vi "Async 985x Incoming Engine.vi"() -> ()   [LabVIEW 2020, in "985x Support Addon Engine.lvlib"]
uses:
  985x Support Addon Engine.lvlib
  <vilib>/NI/NIVS Inline Async API/_VS Inline Async API/Process/Process.lvclass
  Addon/Addon Engine/Types/RT Async Engine Settings.ctl
  Addon/Addon Shared/Types/XNET Settings.ctl
  Frame-Protection-Support/Source/Engine/Types/RT Frame Settings.ctl
  Frame-Protection-Support/Source/Shared/Types/Exported Frame Type.ctl
  Frame-Protection-Support/Source/Engine/Types/RT Protection Configuration.ctl
  Frame-Protection-Support/Source/Shared/Types/Protection Type.ctl
  Frame-Protection-Support/Source/Shared/Types/XNET Signal Configuration.ctl
  Frame-Protection-Support/Source/Shared/Types/Exported Counter Settings.ctl
  Frame-Protection-Support/Source/Shared/Types/Exported Event Trigger Type.ctl
  Frame-Protection-Support/Source/Engine/Types/RT Frame Incoming Values.ctl
  Types/985x Settings.ctl
  Types/FPGA Refnum.ctl
  <vilib>/NI/NIVS Inline Async API/_VS Inline Async API/Process/Process.lvclass/Process.ctl
  <vilib>/NI/NIVS Inline Async API/_VS Inline Async API/Error Handling Process/SubVIs/Error.ConvertArray.vi
  <vilib>/rvi/interface/common/niFpgaWaitOnOcc.vi
  <vilib>/Utility/error.llb/Error Cluster From Error Code.vi
  <vilib>/rvi/errors/niLvFpgaAdjustHostInterfaceError.vi
  985x Properties.vi
  <vilib>/rvi/interface/nirviMethod/nirviMethod.xnode
  <vilib>/rvi/errors/niLvFpgaMergeErrorWithErrorCode.vi
  <vilib>/FPGAPlugInAG/Dynamic/niLvFpga_AcknowledgeIrq_Dynamic.vi
  <vilib>/FPGAPlugInAG/Dynamic/niLvFpga_ReadFifo_Dynamic.vi
  Frame-Protection-Support/Source/Engine/Protection and Counter Support Engine.lvlib
  Frame-Protection-Support/Source/Shared/Protection and Counter Support Shared.lvlib
  Addon/Addon Shared/Protection and Counter Addon Shared.lvlib
  Addon/Addon Engine/Protection and Counter Addon Engine.lvlib
  <vilib>/FPGAPlugInAG/Dynamic/niLvFpga_ConfigureFifo_Dynamic.vi
  <vilib>/FPGAPlugInAG/Dynamic/niLvFpga_StartFifo_Dynamic.vi
panel:
  in  "Parameters":variant
  in  "Process":refnum<class "Process.lvclass">
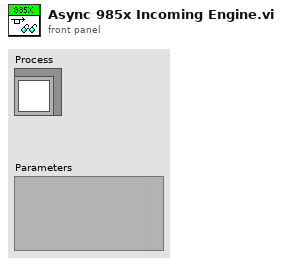
[diagram p1: front panel]
types:
  T1 = enum16{"open", "replace", "create", "open or create", "replace or create", "replace or create with confirmation"}
  T2 = typedef "Protection and Counter Addon Engine.lvlib/RT Async Engine Settings.ctl" = cluster{"Name":string, "Priority":i32, "XNET Settings":T3, "FPGA Session":u32, "Outgoing CAN Session":refnum<k21>, "Outgoing Frame Count":i32, "Outgoing Frames":T4[], "Incoming CAN Session":refnum<k21>, "Incoming Frame Count":i32, "Incoming Frames":T4[], "Incoming Values":T11, "985x Settings":T12}
  T3 = typedef "Protection and Counter Addon Shared.lvlib/XNET Settings.ctl" = cluster{"Database":refnum<k21>, "Cluster":refnum<k21>, "Port":string, "Baud rate [Bd]":u64, "Termination":u32, "CAN I/O Mode":u32, "FD Baud rate [Bd]":u64, "Priority":i32, "Use Legacy":bool, "FD ISO Mode":u32}
  T4 = typedef "Protection and Counter Support Engine.lvlib/RT Frame Settings.ctl" = cluster{"Type":T5, "Frame ID":u32, "Payload Length":u32, "VS Offset":i32, "VS Length":i32, "Frame Conversion":refnum<k21>, "Frame.Data":dbl[], "Generation Period":u32, "Time Since Last Generation":u32, "Generation Iterations":u32, "Generation Counter":u32, "Has Protection?":bool, "Protection Configurations":T6[], "Has Counter?":bool, "Counter Configurations":T9[], "Has Disable?":bool, "Disable VS Index":i32, "Transmit Trigger":T10, "Trigger VS Index":i32}
  T5 = typedef "Protection and Counter Support Shared.lvlib/Exported Frame Type.ctl" = enum16{"Periodic", "Event", "Periodic/Event"}
  T6 = typedef "Protection and Counter Support Engine.lvlib/RT Protection Configuration.ctl" = cluster{"Protection Frame Index":i32, "Protection Type":T7, "Data Indeces":i32[], "Data Array":dbl[], "Check Sum Conversion":refnum<k21>, "CRC Channels":T8[], "Protection VS Index":i32, "Counter Data Index":i32, "Override Index":i32, "Override Value Index":i32}
  T7 = typedef "Protection and Counter Support Shared.lvlib/Protection Type.ctl" = enum16{"Arb ID + Bytes Checksum with Inversion", "Arb ID + Bytes CRC with Inversion", "Reversed Raw Signal Checksum with Inversion", "Concatenated Two's Compliment"}
  T8 = typedef "Protection and Counter Support Shared.lvlib/XNET Signal Configuration.ctl" = cluster{"Start Bit":i32, "Name":string, "Number of bits":i32, "Scale":dbl, "Offset":dbl, "Data Type":u32, "Counter":bool}
  T9 = typedef "Protection and Counter Support Shared.lvlib/Exported Counter Settings.ctl" = cluster{"Frame Index":i32, "Max Count":dbl, "VS Index":i32, "Bit Length":i64, "Override Index":i32, "Override Value Index":i32}
  T10 = typedef "Protection and Counter Support Shared.lvlib/Exported Event Trigger Type.ctl" = enum16{"Channel value change", "Trigger channel (not zero)", "Channel value change or trigger channel (not zero)", "Trigger channel (any value change)", "Channel value change or trigger channel (any value change)"}
  T11 = typedef "Protection and Counter Support Engine.lvlib/RT Frame Incoming Values.ctl" = cluster{"Signal Values":dbl[], "Signal Invalid Values":dbl[], "ProtCtr Sig Values":dbl[], "Timestamps":timestamp[], "Time Differences":dbl[], "IDs":u32[]}
  T12 = typedef "985x Support Addon Engine.lvlib/985x Settings.ctl" = cluster{"Enable":bool, "FPGA Refnum":T13, "Channel Number":u32, "Rx FIFO":refnum<k33>}
  T13 = typedef "985x Support Addon Engine.lvlib/FPGA Refnum.ctl" = refnum<k20>
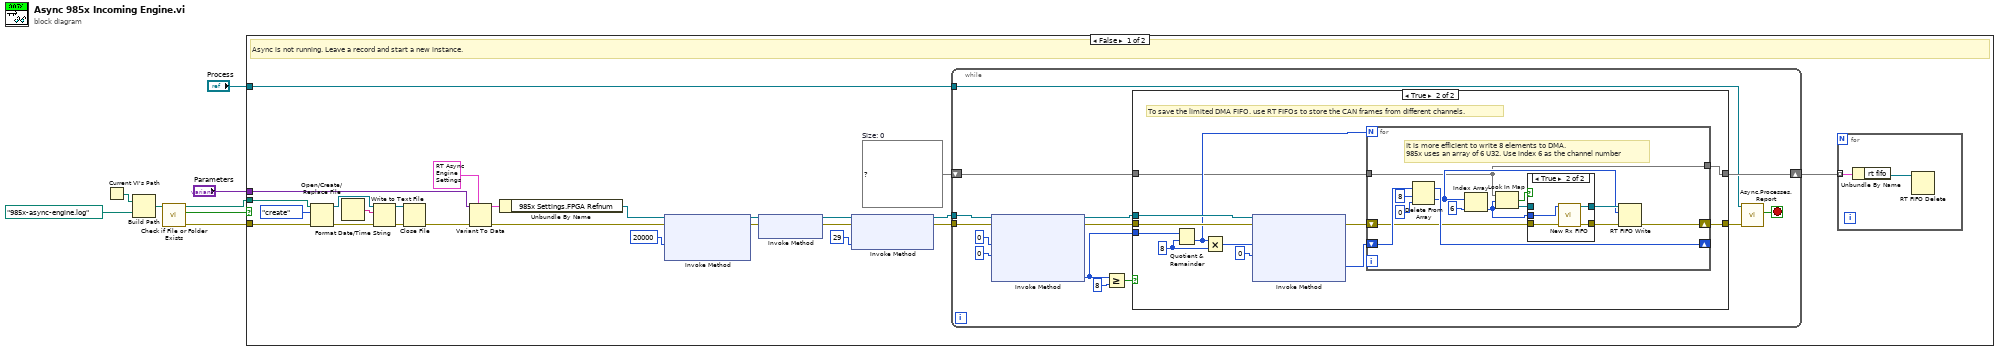
[diagram p0: block diagram]
diagram:
  n1 = Current VI's Path() -> (path=w7:path)
  n2 = Build Path(base path=w7, name or relative path=path "985x-async-engine.log") -> (appended path=w5:path)
  n3 = call <vilib>:"Check if File or Folder Exists.vi"("path"=w5) -> ("error out"=w3:errorcluster, "file or folder exists?"=w2:bool, "dup path"=w4:path)  [unwired: 8 in]
  n4 = case shown="False" w2 {
    tunnel: "Parameters" -> [w23 _]
    tunnel: w4 -> [w14 _]
    tunnel: w3 -> [w13 _]
    tunnel: "Process" -> [w10 _]
    frame False {
      w25 = map{u32, refnum<k33>} {}  # Size: 0
      # "Async is not running. Leave a record and start a new instance."
      n5 = Open/Create/Replace File(file path (use dialog)=w14, error in=w13, operation (0:open)=T1."create") -> (refnum out=w19:refnum<file>, error out=w18:errorcluster)  [unwired: 3 in, 1 out]
      n6 = Format Date/Time String() -> (date/time string=w15:string)  [unwired: 3 in]
      n7 = Write to Text File(file (use dialog)=w19, text=w15, error in=w18) -> (refnum out=w17:refnum<file>, error out=w16:errorcluster)  [unwired: 1 in, 1 out]
      n8 = Close File(refnum=w17, error in=w16) -> (error out=w11:errorcluster)  [unwired: 1 out]
      n9 = Variant To Data(error in=w11, type=T2 {"Name"="", "Priority"=100, "XNET Settings"={"Database"="", "Cluster"="", "Port"="", "Baud rate [Bd]"=0, "Termination"=0, "CAN I/O Mode"=0, "FD Baud rate [Bd]"=500000, "Priority"=100, "Use Legacy"=FALSE, "FD ISO Mode"=0}, "FPGA Session"=0, "Outgoing CAN Session"="", "Outgoing Frame Count"=0, "Outgoing Frames"=[], "Incoming CAN Session"="", "Incoming Frame Count"=0, "Incoming Frames"=[], "Incoming Values"={"Signal Values"=[], "Signal Invalid Values"=[], "ProtCtr Sig Values"=[], "Timestamps"=[], "Time Differences"=[], "IDs"=[]}, "985x Settings"={"Enable"=FALSE, "FPGA Refnum"=refnum, "Channel Number"=0, "Rx FIFO"=refnum}} ("RT Configuration"), Variant=w23) -> (data=w21:T2, error out=w22:errorcluster)
      n10 = Unbundle By Name(w21) -> ("985x Settings.FPGA Refnum"=w20:T13)
      n11 = xnode "Invoke Method"("FPGA VI Reference In"=w20, "error in"=w22, "Requested Depth"=u32 20000) -> ("FPGA VI Reference Out"=w32:T13, "error out"=w31:errorcluster)  [unwired: 1 out]
      n12 = xnode "Invoke Method"("FPGA VI Reference In"=w32, "error in"=w31) -> ("FPGA VI Reference Out"=w30:T13, "error out"=w29:errorcluster)
      n13 = xnode "Invoke Method"("FPGA VI Reference In"=w30, "error in"=w29, "IRQ Number(s)"=29) -> ("FPGA VI Reference Out"=w27:T13, "error out"=w26:errorcluster)
      n14 = while {
        tunnel: w27 -> [w49]
        tunnel: w26 -> [w42]
        shift-right: [w37] -> w9
        shift-left: w25 -> [w40]
        tunnel: w10 -> [w36]
        stop <- w38 stop-if-true
        n15 = xnode "Invoke Method"("FPGA VI Reference In"=w49, "error in"=w42, "Number of Elements"=u32 0, "Timeout (ms)"=0) -> ("FPGA VI Reference Out"=w43:T13, "error out"=w41:errorcluster, "Elements Remaining"=w44:u32)  [unwired: 1 out]
        n16 = Greater Or Equal?(x=w44, y=u32 8) -> (x >= y?=w45:bool)
        n17 = case shown="True" w45 {
          tunnel: w44 -> [_ w60]
          tunnel: w43 -> [_ w58]
          tunnel: w41 -> [w51 w59]
          tunnel: w40 -> [w50 w55]
          tunnel: [w51 w53] -> w39
          tunnel: [w50 w52] -> w37
          frame False {
          }
          frame True {
            w63 = u32 8 ("y")
            # "To save the limited DMA FIFO. use RT FIFOs to store the CAN frames from different channels."
            n18 = Quotient & Remainder(x=w60, y=w63) -> (floor(x/y)=w56:u32)  [unwired: 1 out]
            n19 = Multiply(x=w56, y=w63) -> (x*y=w62:u32)
            n20 = xnode "Invoke Method"("FPGA VI Reference In"=w58, "error in"=w59, "Number of Elements"=w62, "Timeout (ms)"=0) -> ("error out"=w54:errorcluster, "Data"=w57:u32[])  [unwired: 2 out]
            n21 = for {
              N: w56 -> [_]
              shift-right: [w73] -> _
              shift-left: w57 -> [w74]
              tunnel: w55 -> [w64]
              shift-right: [w65] -> w53
              shift-left: w54 -> [w70]
              tunnel: [w64] -> w52
              # "It is more efficient to write 8 elements to DMA.\n985x uses an array of 6 U32. Use index 6 as the channel number"
              n22 = Delete From Array(array=w74, length=8, index=0) -> (deleted portion=w66:u32[], array with subset deleted=w73:u32[])
              n23 = Index Array(array=w66, index=6) -> (element=w71:u32)
              n24 = Look In Map(map=w64, key=w71) -> (key not found?=w72:bool, value=w69:refnum<k33>)  [unwired: 1 in]
              n25 = case shown="True" w72 {
                tunnel: w71 -> [_ w83]
                tunnel: w70 -> [w78 w82]
                tunnel: w69 -> [w79 _]
                tunnel: [w79 w81] -> w68
                tunnel: [w78 w80] -> w67
                frame False {
                }
                frame True {
                  n26 = call "New Rx FIFO.vi"("error in (no error)"=w82, "Channel Number"=w83) -> ("error out"=w80:errorcluster, "Rx FIFO"=w81:refnum<k33>)  [unwired: 8 in]
                }
              }
              n27 = RT FIFO Write(0:w68, 1:w66, 3:w67) -> (11:w65:errorcluster)  [unwired: 2 in, 3 out]
            }
          }
        }
        n28 = call <vilib>:"Async.Processes.Report.vi"("Error"=w39, "Process in"=w36) -> ("Stop"=w38:bool)  [unwired: 8 in, 1 out]
      }
      n29 = for {
        tunnel: w9 -> [w35] mode=indexing
        n30 = Unbundle By Name(w35) -> ("rt fifo"=w34:refnum<k33>)
        n31 = RT FIFO Delete(0:w34) -> ()  [unwired: 2 in, 1 out]
      }
    }
    frame True {
      # "File existed. Async instance has been started. Do nothing."
    }
  }
